vi "VISA(Read).vi"(8 "error in (no error)":errorcluster caption="错误输入（无错误）", 11 "VISA资源名称":refnum<visa-resource-name>) -> (0 "error out":errorcluster caption="错误输出", 1 "F？":bool, 2 "读取缓冲区":string, 3 "VISA资源名称":refnum<visa-resource-name>, 5 "x != 0?":bool)   [LabVIEW 2020, in "人体健康监测系统.lvclass"]
uses:
  b1b6c3e1-e787-4952-aeb8-3e34a96e466b.vi
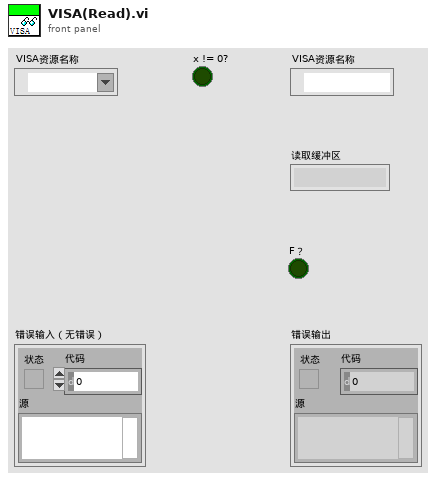
[diagram p1: front panel]
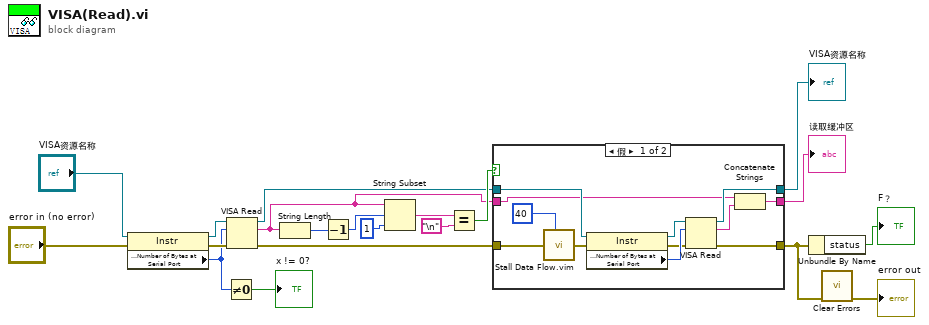
[diagram p0: block diagram]
diagram:
  n1 = property class="Instr"(reference="VISA资源名称", error in="error in (no error)") -> (reference out=w17:refnum<visa-resource-name>, error out=w18:errorcluster, "Serial Settings:Number of Bytes at Serial Port"=w14:u32)
  n2 = Not Equal To 0?(x=w14) -> (x != 0?=→"x != 0?":bool)
  n3 = VISA Read(VISA resource name=w17, byte count=w14, error in (no error)=w18) -> (VISA resource name out=w6:refnum<visa-resource-name>, read buffer=w2:string, error out=w5:errorcluster)  [unwired: 1 out]
  n4 = String Length(string=w2) -> (length=w12:i32)
  n5 = Decrement(x=w12) -> (x-1=w11:i32)
  n6 = String Subset(string=w2, offset (0)=w11, length (rest)=1 ("长度（剩余）")) -> (substring=w9:string)
  n7 = Equal?(x=w9, y="\n") -> (x = y?=w7:bool)
  n8 = case shown="假" w7 {
    tunnel: w6 -> [w29 w35]
    tunnel: w5 -> [w28 w34]
    tunnel: [w27 w34] -> w4
    tunnel: [w26 w35] -> w3
    tunnel: w2 -> [w25 w33]
    tunnel: [w23 w33] -> w1
    frame False {
      n9 = call "Stall Data Flow.vim"("value in"=w28, "milliseconds to wait"=u32 40) -> ("value out"=w22:errorcluster)  [unwired: 1 out]
      n10 = property class="Instr"(reference=w29, error in=w22) -> (reference out=w31:refnum<visa-resource-name>, error out=w30:errorcluster, "Serial Settings:Number of Bytes at Serial Port"=w32:u32)
      n11 = VISA Read(VISA resource name=w31, byte count=w32, error in (no error)=w30) -> (VISA resource name out=w26:refnum<visa-resource-name>, read buffer=w24:string, error out=w27:errorcluster)  [unwired: 1 out]
      n12 = Concatenate Strings(w25, w24) -> (w23:string)
    }
    frame True {
    }
  }
  "VISA资源名称" <- w3
  "读取缓冲区" <- w1
  n13 = Unbundle By Name(w4) -> ("status"=→"F？":bool)
  n14 = call <vilib>:"Clear Errors.vi"("error in (no error)"=w4) -> ("error out"=→"error out":errorcluster)  [unwired: 5 in, 1 out]
